vi "MIU_LeakTest_v1.1.vi"() -> ()   [LabVIEW 2010]
uses:
  <vilib>/Utility/error.llb/DialogType.ctl
  <vilib>/Instr/_visa.llb/VISA Configure Serial Port (Instr).vi
  <vilib>/Analysis/NI_AALPro.lvlib
panel:
  out "Current Valve":dbl
  in  "stop":bool
  in  "Switching Delay":dbl=5000.0
  in  "Offset in Serial":i32=190
  out "PRESSURE":string="0"
  out "PRESSURE":dbl(graph)=80.268
  in  "Control Port":refnum<visa-resource-name>="COM4"
  in  "Control baud rate":u32=9600
  out "Time":string="0"
  out "Date":string="0"
  in  "Serial Read Port":refnum<visa-resource-name>="COM5"
  in  "data bits":u16=8 min=5 max=8 step=1
  in  "parity":u16(ring) items=["None", "Odd", "Even", "Mark", "Space"]
  in  "stop bits":u16(ring)=10 items=["1.0"=10, "1.5"=15, "2.0"=20]
  in  "flow control":u16(ring) items=["None"=0, "XON/XOFF"=1, "RTS/CTS"=2, "DTR/DSR"=4]
  in  "byte count":u32=500
  out "return count":u32
  in  "Instrument baud rate (9600)":u32=9600
  out "Pressure Leak Rate":cluster{i32[], "Best Linear Fit":dbl[]}[](graph)
  out "Leak Rate":dbl
  in  "Points to Average":i32=30
  # "N2O/CO: 190"
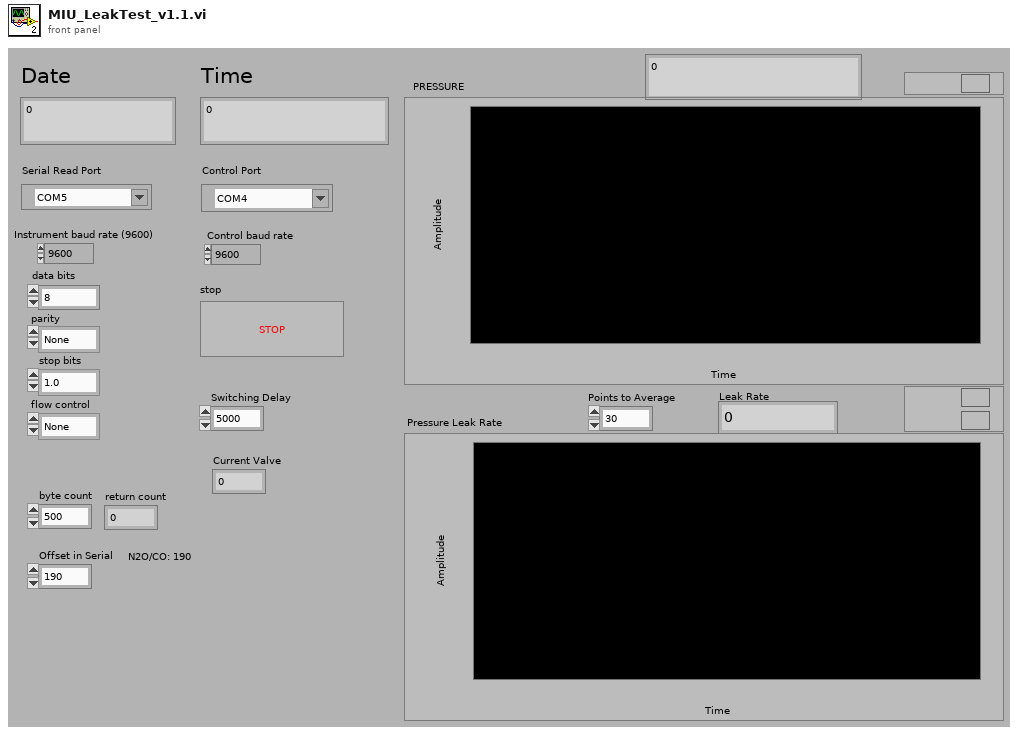
[diagram p1: front panel]
types:
  T1 = typedef "DialogType.ctl" = u16
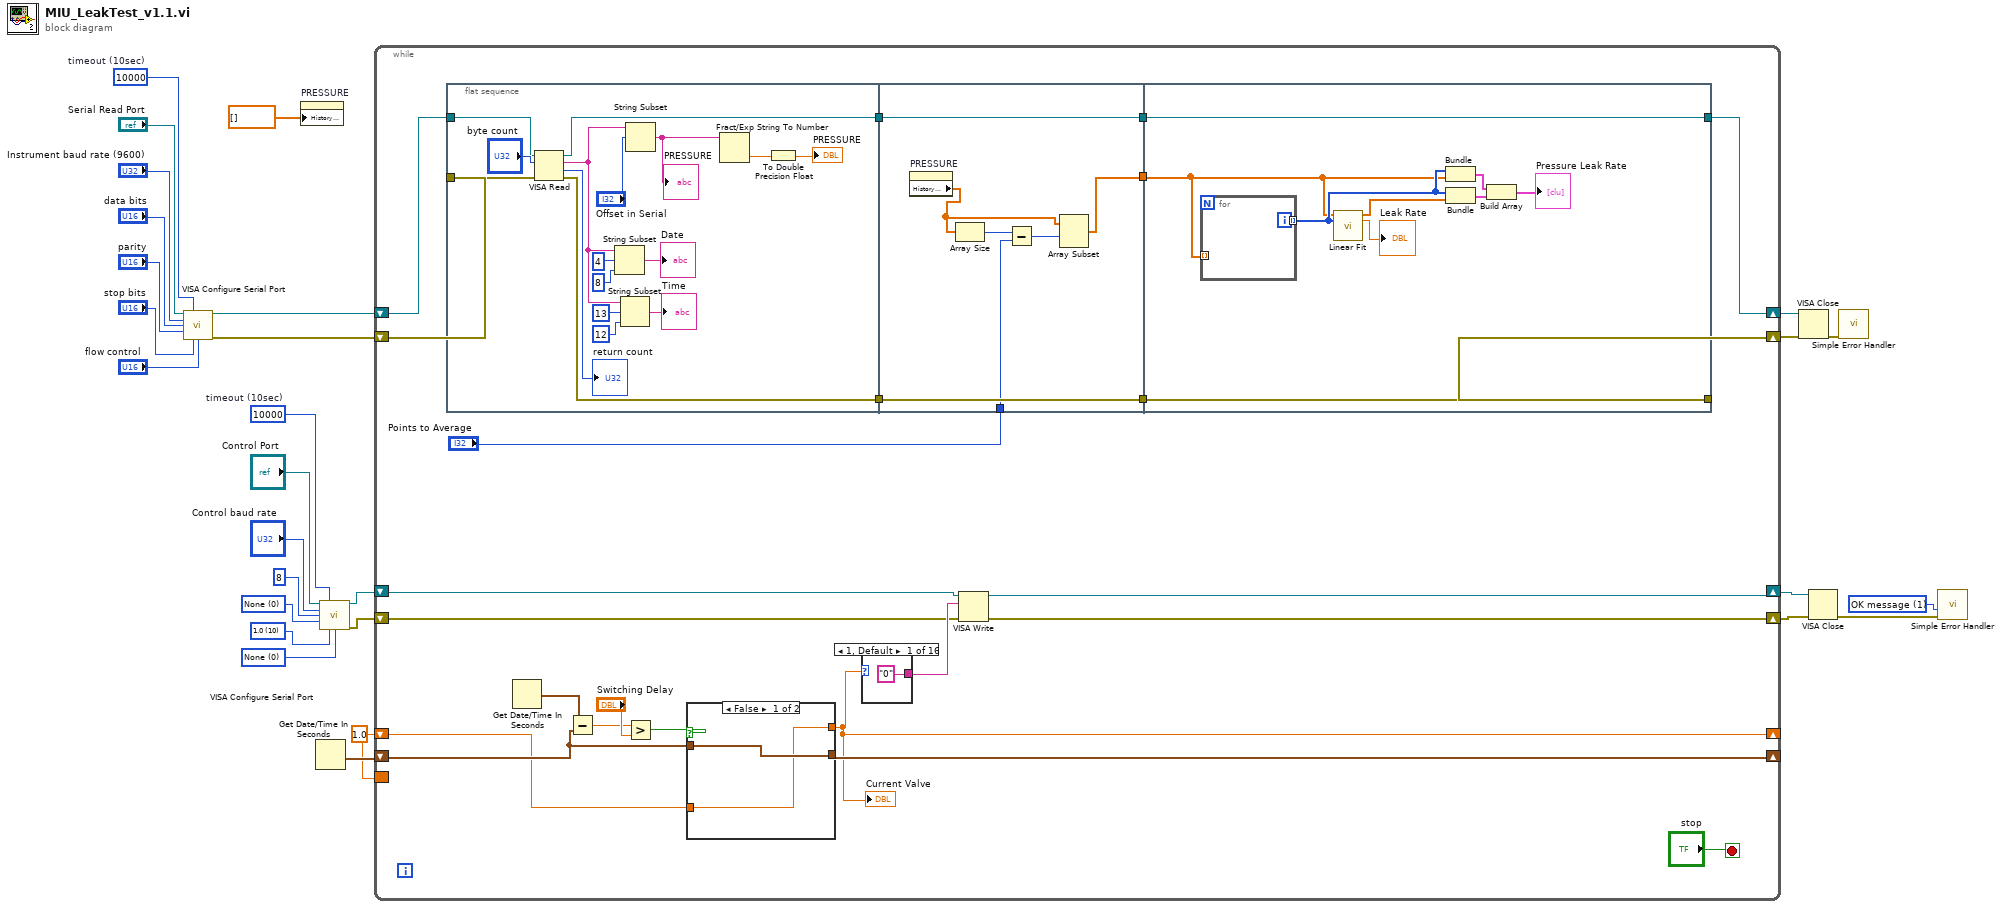
[diagram p0: block diagram]
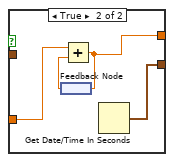
[diagram p2: hidden frame]
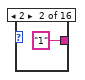
[diagram p3: hidden frame]
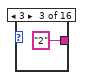
[diagram p4: hidden frame]
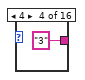
[diagram p5: hidden frame]
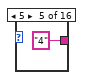
[diagram p6: hidden frame]
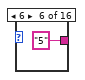
[diagram p7: hidden frame]
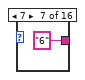
[diagram p8: hidden frame]
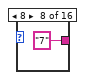
[diagram p9: hidden frame]
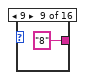
[diagram p10: hidden frame]
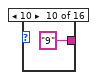
[diagram p11: hidden frame]
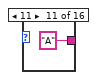
[diagram p12: hidden frame]
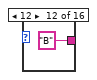
[diagram p13: hidden frame]
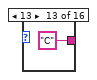
[diagram p14: hidden frame]
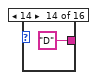
[diagram p15: hidden frame]
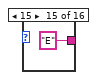
[diagram p16: hidden frame]
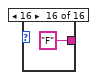
[diagram p17: hidden frame]
diagram:
  w5 = 1.0
  w9 = T1 1 items=["no dialog", "OK message", "continue or stop message", "OK message + warnings", "continue/stop + warnings"] ("type of dialog (OK msg:1)")
  w13 = u16 0 items=["None"=0, "XON/XOFF"=1, "RTS/CTS"=2, "DTR/DSR"=4] ("flow control")
  w14 = u16 10 items=["1.0"=10, "1.5"=15, "2.0"=20] ("stop bits")
  w16 = u16 0 items=["None", "Odd", "Even", "Mark", "Space"] ("parity")
  w15 = u32 10000  # timeout (10sec)
  w25 = u32 10000  # timeout (10sec)
  n1 = call-poly "VISA Configure Serial Port"("VISA resource name"="Serial Read Port", "timeout (10sec)"=w25, "baud rate (9600)"="Instrument baud rate (9600)", "data bits (8)"="data bits", "parity (0:none)"="parity", "stop bits (10: 1 bit)"="stop bits", "flow control (0:none)"="flow control") -> ("VISA resource name out"=w8:refnum<visa-resource-name>, "error out"=w7:errorcluster)  [unwired: 2 in, 5 out]
  n2 = property on="PRESSURE" class="WFChart (strict)"("History Data"=dbl[] []) -> ()  [unwired: 2 in, 2 out]
  n3 = Get Date/Time In Seconds() -> (seconds since 1Jan1904=w6:timestamp)
  n4 = call-poly "VISA Configure Serial Port"("VISA resource name"="Control Port", "timeout (10sec)"=w15, "baud rate (9600)"="Control baud rate", "data bits (8)"=u16 8 ("data bits"), "parity (0:none)"=w16, "stop bits (10: 1 bit)"=w14, "flow control (0:none)"=w13) -> ("VISA resource name out"=w4:refnum<visa-resource-name>, "error out"=w3:errorcluster)  [unwired: 2 in, 5 out]
  n5 = while {
    shift-right: [w52] -> w21
    shift-left: w8 -> [w49]
    shift-right: [w51] -> w20
    shift-left: w7 -> [w50]
    shift-right: [w36] -> _
    shift-left: w6 -> [w37]
    border: w5 -> [_]
    shift-right: [w34] -> _
    shift-left: w5 -> [w35]
    shift-right: [w31] -> w2
    shift-left: w4 -> [w33]
    shift-right: [w30] -> w1
    shift-left: w3 -> [w32]
    stop <- "stop" stop-if-true
    n6 = flat-sequence {
      tunnel: w50 -> [w77]
      tunnel: w49 -> [w76]
      tunnel: [w85] -> w48
      tunnel: [w79] -> w47
      tunnel: w48 -> [w98]
      tunnel: w47 -> [w97]
      tunnel: "Points to Average" -> [w93]
      tunnel: [w98] -> w45
      tunnel: [w97] -> w44
      tunnel: [w92] -> w43
      tunnel: [w106] -> w51
      tunnel: [w107] -> w52
      tunnel: w45 -> [w107]
      tunnel: w44 -> [w106]
      tunnel: w43 -> [w99]
      frame #0 {
        n7 = VISA Read(VISA resource name=w76, byte count="byte count", error in (no error)=w77) -> (VISA resource name out=w85:refnum<visa-resource-name>, read buffer=w81:string, return count=→"return count":u32, error out=w79:errorcluster)
        n8 = String Subset(string=w81, offset (0)=4, length (rest)=8 ("length (rest)")) -> (substring=→"Date":string)
        n9 = String Subset(string=w81, offset (0)=13, length (rest)=12 ("length (rest)")) -> (substring=→"Time":string)
        n10 = String Subset(string=w81, offset (0)="Offset in Serial") -> (substring=w82:string)  [unwired: 1 in]
        "PRESSURE" <- w82
        n11 = Fract/Exp String To Number(string=w82) -> (number=w83:dbl)  [unwired: 3 in, 1 out]
        n12 = To Double Precision Float(number=w83) -> (double precision float=→"PRESSURE":dbl)
      }
      frame #1 {
        n13 = property on="PRESSURE" class="WFChart (strict)"() -> ("History Data"=w94:dbl[])  [unwired: 2 in, 2 out]
        n14 = Array Size(array=w94) -> (size(s)=w95:i32)
        n15 = Subtract(x=w95, y=w93) -> (x-y=w96:i32)
        n16 = Array Subset(array=w94, index=w96) -> (w92:dbl[])  [unwired: 1 in]
      }
      frame #2 {
        n17 = for {
          tunnel: [w108] -> w105 mode=indexing
          tunnel: w99 -> [_] mode=indexing
          i -> [w108]
        }
        n18 = call <vilib>:"Linear Fit.vi"("Y"=w99, "X"=w105) -> ("Best Linear Fit"=w104:dbl[], "slope"=→"Leak Rate":dbl)  [unwired: 9 in, 3 out]
        n19 = Bundle(w105, w99) -> (w103:cluster{i32[], dbl[]})  [unwired: 1 in]
        n20 = Bundle(w105, "Best Linear Fit"=w104) -> (w102:cluster{i32[], "Best Linear Fit":dbl[]})  [unwired: 1 in]
        n21 = Build Array(w103, w102) -> (→"Pressure Leak Rate":cluster{i32[], "Best Linear Fit":dbl[]}[])
      }
    }
    n22 = Get Date/Time In Seconds() -> (seconds since 1Jan1904=w39:timestamp)
    n23 = Subtract(x=w39, y=w37) -> (x-y=w40:dbl)
    n24 = Greater?(x=w40, y="Switching Delay") -> (0:w42:bool)
    n25 = case shown="False" w42 {
      tunnel: [w54 w58] -> w36
      tunnel: w37 -> [w54 _]
      tunnel: [w53 w56] -> w34
      tunnel: w35 -> [w53 w55]
      frame False {
      }
      frame True {
        n26 = feedback #1() -> (w57:dbl)
        n27 = Add(x=w55, y=w57) -> (x+y=w56:dbl)
        n28 = feedback-in #1(w56) -> ()
        n29 = Get Date/Time In Seconds() -> (seconds since 1Jan1904=w58:timestamp)
      }
    }
    "Current Valve" <- w34
    n30 = case shown="1, Default" w34 {
      tunnel: ["0" "1" "2" "3" "4" "5" "6" "7" "8" "9" "A" "B" "C" "D" "E" "F"] -> w38
      frame 1, Default {
      }
      frame 2 {
      }
      frame 3 {
      }
      frame 4 {
      }
      frame 5 {
      }
      frame 6 {
      }
      frame 7 {
      }
      frame 8 {
      }
      frame 9 {
      }
      frame 10 {
      }
      frame 11 {
      }
      frame 12 {
      }
      frame 13 {
      }
      frame 14 {
      }
      frame 15 {
      }
      frame 16 {
      }
    }
    n31 = VISA Write(VISA resource name=w33, write buffer=w38, error in (no error)=w32) -> (VISA resource name out=w31:refnum<visa-resource-name>, error out=w30:errorcluster)  [unwired: 1 out]
  }
  n32 = VISA Close(VISA resource name=w21, error in (no error)=w20) -> (error out=w27:errorcluster)
  n33 = VISA Close(VISA resource name=w2, error in (no error)=w1) -> (error out=w11:errorcluster)
  n34 = call <vilib>:"Simple Error Handler.vi"("error in (no error)"=w27) -> ()  [unwired: 1 in, 8 out]
  n35 = call <vilib>:"Simple Error Handler.vi"("type of dialog (OK msg:1)"=w9, "error in (no error)"=w11) -> ()  [unwired: 8 out]
